vi "Test.vi"() -> ()   [LabVIEW 2020, in "PNS.lvlib"]
uses:
  PNS.lvlib
  Seiten/CalGas Aufschaltung/FGV CalGas Aktionen.ctl
  Seiten/CalGas Aufschaltung/Auswahl Aufschaltpunkt.ctl
  Seiten/CalGas Aufschaltung/CalGas Aufschaltung.lvlib
panel:
  in  "Aktion":enum16{"lesen", "prüfen"}(ring)
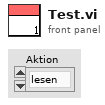
[diagram p1: front panel]
types:
  T1 = typedef "CalGas Aufschaltung.lvlib/FGV CalGas Aktionen.ctl" = enum16{"lesen", "Def.CalGas", "Aufschaltung CalGas", "laden", "speichern", "KAL extrahieren"}
  T2 = typedef "CalGas Aufschaltung.lvlib/Auswahl Aufschaltpunkt.ctl" = enum16{"über Filterblock", "Analysator direkt", "über PNS", "Entnahme"}
  T3 = typedef "CalGas Aufschaltung.lvlib/Aufschaltung CalGas.ctl" = cluster{"Kalibriergas":T4, "Aufschaltpunkt":T2, "Analysator":T5}
  T4 = typedef "Auswahlfeld.ctl" = u16
  T5 = typedef "CalGas Aufschaltung.lvlib/Auswahl Analysator.ctl" = enum16{"FT-IR", "FID", "PMA", "PMA/FID/FT-IR"}
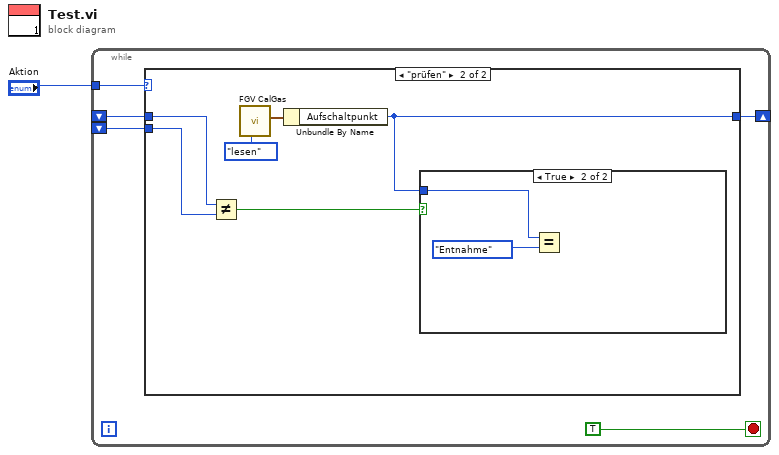
[diagram p0: block diagram]
diagram:
  n1 = while {
    shift-right: [w5] -> _
    shift-left: _ -> [w4]
    tunnel: "Aktion" -> [w3]
    shift-left: _ -> [w2]
    stop <- TRUE stop-if-true
    n2 = case shown="\"prüfen\"" w3 {
      tunnel: [w7 w8] -> w5
      tunnel: w4 -> [w7 w11]
      tunnel: w2 -> [_ w10]
      frame "lesen", Default {
      }
      frame "prüfen" {
        n3 = Not Equal?(x=w11, y=w10) -> (x != y?=w9:bool)
        n4 = call "FGV CalGas.vi"("Aktionen"=FGV_CalGas_Aktionen."lesen") -> ("Aufschaltung CalGas"=w12:T3)  [unwired: 7 in, 3 out]
        n5 = Unbundle By Name(w12) -> ("Aufschaltpunkt"=w8:T2)
        n6 = case shown="True" w9 {
          tunnel: w8 -> [_ w14]
          frame False {
          }
          frame True {
            n7 = Equal?(x=w14, y=Auswahl_Aufschaltpunkt."Entnahme") -> ()  [unwired: 1 out]
          }
        }
      }
    }
  }
